vi "ort_find_max.vi"(6 "inputValid":bool, 8 "endOfCycle":bool, 10 "ort.p.methodParams":T1, 11 "data":cluster{"index":u16, "data":i16}) -> (0 "outputValid":bool, 1 "cycleMaxMonitor":fxp<+/-,24,16>, 2 "maxIndex":u16, 3 "cycleMax":fxp<+/-,24,16>)   [LabVIEW 2016]
uses:
  <instrlib>/_niInstr/Basic Elements/v1/FPGA/niInstr Basic Elements v1 FPGA.lvlib
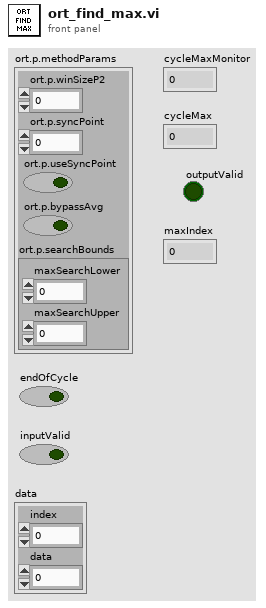
[diagram p1: front panel]
types:
  T1 = cluster{"ort.p.winSizeP2":u16, "ort.p.syncPoint":u16, "ort.p.useSyncPoint":bool, "ort.p.bypassAvg":bool, "ort.p.searchBounds":cluster{"maxSearchLower":u16, "maxSearchUpper":u16}}
  T2 = cluster{"maxSearchLower":u16, "maxSearchUpper":u16}
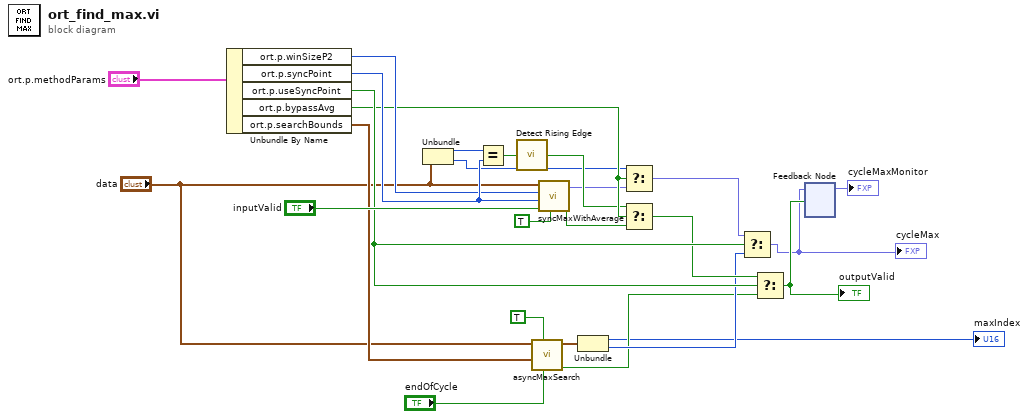
[diagram p0: block diagram]
diagram:
  n1 = Unbundle By Name("ort.p.methodParams") -> ("ort.p.winSizeP2"=w22:u16, "ort.p.syncPoint"=w23:u16, "ort.p.useSyncPoint"=w24:bool, "ort.p.bypassAvg"=w21:bool, "ort.p.searchBounds"=w25:T2)
  n2 = Unbundle("data") -> ("index"=w5:u16, "data"=w7:i16)
  n3 = Equal?(x=w5, y=w23) -> (x = y?=w6:bool)
  n4 = call <instrlib>:"Detect Rising Edge.vi"("signal"=w6) -> ("edge detected"=w8:bool)  [unwired: 14 in]
  n5 = call "asyncMaxSearch.vi"("reset"="endOfCycle", "enable"=TRUE, "maxSearchBounds"=w25, "inputPair"="data") -> ("outputValid"=w9:bool, "output"=w2:cluster{"index":u16, "data":i16})  [unwired: 6 in]
  n6 = call "syncMaxWithAverage.vi"("enable"=TRUE, "inputValid"="inputValid", "syncPoint"=w23, "syncAverageBand"=w22, "input"="data") -> ("outputValid"=w4:bool, "waveMaxAvg"=w1:fxp<+/-,24,16>)  [unwired: 5 in]
  n7 = Unbundle(w2) -> ("index"=→"maxIndex":u16, "data"=w10:i16)
  n8 = Select(t=w7, s=w21, f=w1) -> (s? t:f=w12:fxp<+/-,24,16>)
  n9 = Select(t=w8, s=w21, f=w4) -> (s? t:f=w11:bool)
  n10 = Select(t=w12, s=w24, f=w10) -> (s? t:f=w16:fxp<+/-,24,16>)
  "cycleMax" <- w16
  n11 = Select(t=w11, s=w24, f=w9) -> (s? t:f=w17:bool)
  "outputValid" <- w17
  n12 = feedback #1() -> (→"cycleMaxMonitor":fxp<+/-,24,16>)  [unwired: 1 in]
  n13 = feedback-in #1(w16, w17) -> ()
